vi "Encoder Conversions.vi"(9 "Distance (ft)":dbl, 11 "Encoder Counts Per Distance":dbl) -> (1 "Encoder Counts Per Distance":dbl, 2 "Distance (Feet)":dbl, 3 "Distance (in)":dbl)   [LabVIEW 2018]
uses:
  Infrastructure/Constants.vi
panel:
  in  "Distance (in)":dbl
  # "encoder counts ----> distance"
  # "formula: distance {ft} = [(encoder counts per distance * wheel diameter)/ (encoder counts per rotation * pi)] / 12"
  # "distance ----> encoder counts"
  # "formula: encoder counts per distance = (distance/wheel diameter) * pi * encoder counts per rotation"
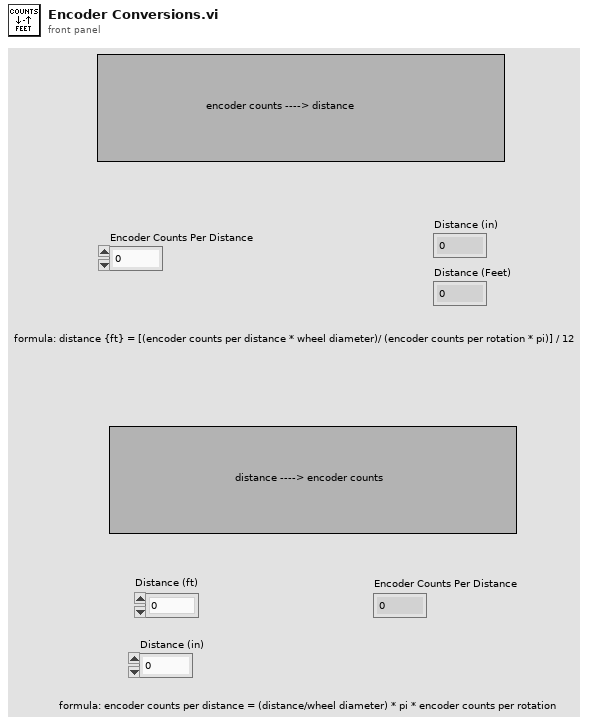
[diagram p1: front panel]
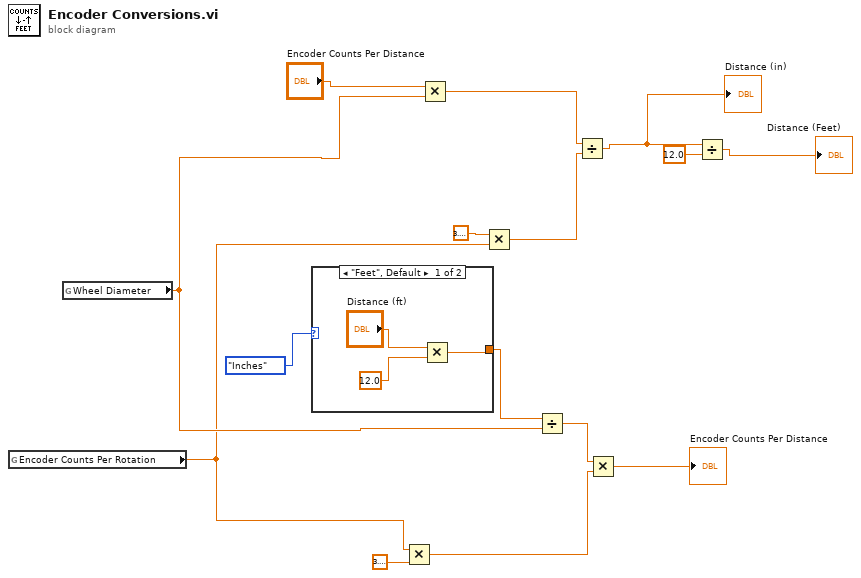
[diagram p0: block diagram]
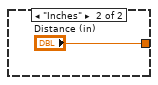
[diagram p2: hidden frame]
diagram:
  n1 = global read "Constants.vi" "Encoder Counts Per Rotation"() -> (w3:dbl)
  n2 = global read "Constants.vi" "Wheel Diameter"() -> (w4:dbl)
  n3 = case shown="\"Feet\", Default" enum16{"Feet", "Inches"}."Inches" {
    tunnel: [w16 "Distance (in)"] -> w1
    frame "Feet", Default {
      n4 = Multiply(x="Distance (ft)", y=12.0) -> (x*y=w16:dbl)
    }
    frame "Inches" {
    }
  }
  n5 = Multiply(x=w3, y=3.141592653589793) -> (x*y=w14:dbl)
  n6 = Multiply(x="Encoder Counts Per Distance", y=w4) -> (x*y=w9:dbl)
  n7 = Multiply(x=3.141592653589793, y=w3) -> (x*y=w10:dbl)
  n8 = Divide(x=w1, y=w4) -> (x/y=w13:dbl)
  n9 = Divide(x=w9, y=w10) -> (x/y=w12:dbl)
  "Distance (in)" <- w12
  n10 = Multiply(x=w13, y=w14) -> (x*y=→"Encoder Counts Per Distance":dbl)
  n11 = Divide(x=w12, y=12.0) -> (x/y=→"Distance (Feet)":dbl)
